vi "BonOMM-SAOMM.vi"() -> ()   [LabVIEW 2019] (continued)
                n1946 = local write "RangeTable"(FALSE ("RangeTable")) -> ()
                n1947 = case shown="Vrai" w5739 {
                  frame False {
                  }
                  frame True {
                    n1948 = local read "LimXPesto"() -> (w5740:dbl)
                    n1949 = local read "BrasPesto"() -> (w5741:bool)
                    n1950 = local read "Table VRN"() -> (w5750:refnum<visa-resource-name>)
                    n1951 = local read "Table Error"() -> (w5748:errorcluster)
                    n1952 = control-ref of="TERMINAL"() -> (w5753:refnum<vi>)
                    n1953 = control-ref of="Indicateur d'état"() -> (w5752:refnum<vi>)
                    n1954 = control-ref of="Table actif"() -> (w5745:refnum<vi>)
                    n1955 = call "Newmark-GotoAll.vi"("Table VRN IN"=w5750, "BrasPesto"=w5741, "Bool Refnum"=w5745, "LimXPesto"=w5740, "Notify?"=FALSE, "Error IN"=w5748, "Position X"="Rangement Y", "Position Y"="Rangement X", "Position Z"="Rangement Z") -> ("Table VRN OUT"=w5749:refnum<visa-resource-name>, "Error OUT"=w5747:errorcluster)  [unwired: 5 in]
                    n1956 = call "TERMINAL.vi"("Indicateur Refnum"=w5752, "Terminal Refnum"=w5753, "Indicateur d'état"="Commande de rangement des tables") -> ()
                    n1957 = local write "Table VRN"(w5749) -> ()
                    n1958 = local write "Table Error"(w5747) -> ()
                    n1959 = local write "Cible X"("Rangement Y") -> ()
                    n1960 = local write "Cible Y"("Rangement X") -> ()
                    n1961 = local write "Cible Z"("Rangement Z") -> ()
                  }
                }
              }
              event "GO": Value Change {
                n1962 = event-data() -> ()  [unwired: 1 in, 5 out]
                n1963 = flat-sequence {
                  frame #0 {
                    n1964 = control-ref of="TERMINAL"() -> (w5756:refnum<vi>)
                    n1965 = control-ref of="Indicateur d'état"() -> (w5755:refnum<vi>)
                    n1966 = local write "GO"(FALSE) -> ()
                    n1967 = call "TERMINAL.vi"("Indicateur Refnum"=w5755, "Terminal Refnum"=w5756, "Indicateur d'état"="Commande de déplacement du télescope") -> ()
                  }
                  frame #1 {
                    n1968 = local read "STATH"() -> (w5758:bool[])
                    n1969 = Index Array(array=w5758, index=7 ("Index")) -> (element=w5759:bool)
                    n1970 = case shown="Vrai" w5759 {
                      frame False {
                        w5761 = u32 0
                        # "Est-ce qu'on ne veut pas envoyez un stop à ce moment là ?"
                        n1971 = local read "FIFO d'erreur"() -> (w5763:T7)
                        n1972 = Bundle("TCS", w5761, w5761, "ATTENTION!!\nLes moteurs ne sont pas allumés.") -> (w5764:cluster{string, u32, u32, string})  [unwired: 1 in]
                        n1973 = Build Array (concatenate)(w5763, w5764) -> (w5762:T7)
                        n1974 = local write "FIFO d'erreur"(w5762) -> ()
                      }
                      frame True {
                        n1975 = control-ref of="TCS actif"() -> (w5767:refnum<vi>)
                        n1976 = local read "TCS VRN"() -> (w5768:refnum<visa-resource-name>)
                        n1977 = call "EXCOM-CMD.vi"("VRN IN"=w5768, "Bool Refnum"=w5767, "Commande #"=12) -> ("VRN OUT"=w5771:refnum<visa-resource-name>, "OK Done"=w5770:bool, "Error OUT"=w5769:errorcluster)  [unwired: 10 in]
                        n1978 = local write "TCS VRN"(w5771) -> ()
                        n1979 = local write "TCS Error"(w5769) -> ()
                        n1980 = case shown="Vrai" w5770 {
                          selector: w5770 -> [_ w5775]
                          frame False {
                            n1981 = One Button Dialog(message="ATTENTION!!\nProblème de communication\navec TCS-Ctrl", button name ("OK")="OK" ("nom du bouton (\"OK\")")) -> ()  [unwired: 1 out]
                          }
                          frame True {
                            "Déplacement usager" <- w5775
                          }
                        }
                      }
                    }
                  }
                }
              }
              event "Synctel": Value Change {
                n1982 = event-data() -> ()  [unwired: 1 in, 5 out]
                n1983 = local read "Mode Est"() -> (w5776:bool)
                n1984 = case shown="Faux" w5776 {
                  frame False {
                    n1985 = flat-sequence {
                      frame #0 {
                        n1986 = local write "Synctel"(FALSE) -> ()
                      }
                      frame #1 {
                        w5781 = ", " ("F button name (\"Cancel\")")
                        n1987 = local read "NO epoch"() -> (w5787:dbl)
                        n1988 = local read "N.O. A.D."() -> (w5783:string)
                        n1989 = local read "N.O. Déc."() -> (w5780:string)
                        n1990 = Number To Fractional String(number=w5787, width (-)=i16 6, precision (6)=i16 2) -> (F-format string=w5779:string)  [unwired: 1 in]
                        n1991 = Concatenate Strings("êtes vous certain de vouloir synchroniser \nles coordonnées de TCS sur :\nR.A. : " ("string"), w5783, "\nDEC : ", w5780, "\nEPOCH : ", w5779) -> (w5791:string)
                        n1992 = control-ref of="TERMINAL"() -> (w5785:refnum<vi>)
                        n1993 = control-ref of="Indicateur d'état"() -> (w5784:refnum<vi>)
                        n1994 = Concatenate Strings("Synchronisation sur : " ("Indicateur d'état"), w5783, w5781, w5780, w5781, w5779) -> (w5778:string)
                        n1995 = Two Button Dialog(message=w5791, 1:"NON" ("F button name (\"Cancel\")"), 2:"OUI" ("T button name (\"OK\")")) -> (T button?=w5793:bool)
                        n1996 = call "TERMINAL.vi"("Indicateur Refnum"=w5784, "Terminal Refnum"=w5785, "Indicateur d'état"=w5778) -> ()
                        n1997 = case shown="Vrai" w5793 {
                          tunnel: w5780 -> [_ w5807]
                          tunnel: w5783 -> [_ w5806]
                          frame False {
                          }
                          frame True {
                            # "Initialise RA et DEC\naux valeurs de Starry Night"
                            n1998 = local read "NO epoch"() -> (w5803:dbl)
                            n1999 = call "time-str-to-time-dbl-RA.vi"("Chaîne"=w5806) -> ("TCS_coords"=w5801:dbl)
                            n2000 = call "time-str-to-time-dbl-DEC.vi"("Chaîne"=w5807) -> ("TCS_coords"=w5802:dbl)
                            n2001 = control-ref of="TCS actif"() -> (w5796:refnum<vi>)
                            n2002 = local read "TCS VRN"() -> (w5804:refnum<visa-resource-name>)
                            n2003 = Build Array(w5801, w5802, w5803) -> (w5800:dbl[])
                            n2004 = call "EXCOM-CMD.vi"("VRN IN"=w5804, "Bool Refnum"=w5796, "Commande #"=3 ("NombredArguments"), "Args"=w5800) -> ("VRN OUT"=w5797:refnum<visa-resource-name>, "OK Done"=w5798:bool, "Error OUT"=w5799:errorcluster)  [unwired: 9 in]
                            n2005 = local write "TCS Error"(w5799) -> ()
                            n2006 = local write "TCS VRN"(w5797) -> ()
                            n2007 = case shown="Faux" w5798 {
                              frame False {
                                n2008 = One Button Dialog(message="ATTENTION!!\nLa commande SyncTEL a échoué.\nVérifiez TCS.", button name ("OK")="OK" ("nom du bouton (\"OK\")")) -> ()  [unwired: 1 out]
                              }
                              frame True {
                              }
                            }
                          }
                        }
                      }
                      frame #2 {
                        n2009 = control-ref of="TCS actif"() -> (w5810:refnum<vi>)
                        n2010 = local read "TCS VRN"() -> (w5812:refnum<visa-resource-name>)
                        n2011 = local read "TCS Error"() -> (w5811:errorcluster)
                        n2012 = call "EXCOM-CMD.vi"("VRN IN"=w5812, "Bool Refnum"=w5810, "Commande #"=13 ("NombredArguments"), "Error IN"=w5811) -> ("VRN OUT"=w5814:refnum<visa-resource-name>, "Error OUT"=w5813:errorcluster)  [unwired: 9 in, 1 out]
                        n2013 = local write "TCS VRN"(w5814) -> ()
                        n2014 = local write "TCS Error"(w5813) -> ()
                      }
                    }
                  }
                  frame True {
                    n2015 = One Button Dialog(message="Impossible de synchroniser les coordonnées en mode inversé.", button name ("OK")="Ok") -> ()  [unwired: 1 out]
                  }
                }
              }
              event "RotationTCS": Value Change {
                n2016 = event-data() -> ()  [unwired: 1 in, 5 out]
              }
              event "ModifRotation": Value Change {
                n2017 = event-data() -> ()  [unwired: 1 in, 5 out]
                n2018 = case shown="Vrai" "ModifRotation" {
                  frame False {
                  }
                  frame True {
                    n2019 = local read "RotationTCS"() -> (w5826:dbl)
                    n2020 = control-ref of="TCS actif"() -> (w5819:refnum<vi>)
                    n2021 = local read "TCS VRN"() -> (w5823:refnum<visa-resource-name>)
                    n2022 = call "Set rotation.vi"("Rot.In"=w5826) -> ("DONE"=w5825:bool, "Rot.Out"=w5824:dbl)
                    n2023 = case shown="Vrai" w5825 {
                      selector: w5825 -> [w5827 _]
                      tunnel: w5824 -> [_ w5830]
                      tunnel: w5823 -> [_ w5834]
                      tunnel: w5819 -> [_ w5833]
                      frame False {
                        n2024 = local write "ModifRotation"(w5827) -> ()
                      }
                      frame True {
                        n2025 = In Range and Coerce(upper limit=180.0, x=w5830, lower limit=0.0 ("upper limit")) -> (coerced(x)=w5828:dbl, In Range?=w5829:bool)
                        n2026 = case shown="Vrai" w5829 {
                          tunnel: w5834 -> [_ w5839]
                          tunnel: w5833 -> [_ w5838]
                          tunnel: w5828 -> [_ w5836]
                          frame False {
                            n2027 = One Button Dialog(message="Les valeurs envoyées doivent être comprises entre 0° et 180°") -> ()  [unwired: 1 in, 1 out]
                          }
                          frame True {
                            # "Bug TCS"
                            n2028 = expression code="90-x"(w5836) -> (w5837:dbl)
                            n2029 = stacked-sequence {
                              tunnel: w5837 -> [_ w5845 _]
                              tunnel: w5839 -> [_ w5849 _]
                              tunnel: w5838 -> [_ w5843 _]
                              frame #0 {
                                w5841 = 2
                                w5840 = 2
                                # "Attendre 0.5 sec afin que la boucle de surveillance se termine"
                                n2030 = property on="ModifRotation" class="Bool (strict)"("Blinking"=TRUE) -> ()  [unwired: 2 in, 2 out]
                                n2031 = property on="GO" class="Bool (strict)"("Disabled"=w5840) -> ()  [unwired: 2 in, 2 out]
                                n2032 = property on="ModCoor" class="Bool (strict)"("Disabled"=w5840) -> ()  [unwired: 2 in, 2 out]
                                n2033 = property on="Synctel" class="Bool (strict)"("Disabled"=w5840) -> ()  [unwired: 2 in, 2 out]
                                n2034 = property on="Offset OK" class="Bool (strict)"("Disabled"=w5840) -> ()  [unwired: 2 in, 2 out]
                                n2035 = property on="Zénith" class="Bool (strict)"("Disabled"=w5841) -> ()  [unwired: 2 in, 2 out]
                                n2036 = property on="Écran" class="Bool (strict)"("Disabled"=w5841) -> ()  [unwired: 2 in, 2 out]
                                n2037 = property on="ModifFoyer" class="Bool (strict)"("Disabled"=w5841) -> ()  [unwired: 2 in, 2 out]
                                n2038 = property on="Range" class="Bool (strict)"("Disabled"=w5841) -> ()  [unwired: 2 in, 2 out]
                                n2039 = property on="ModifDome" class="Bool (strict)"("Disabled"=w5841) -> ()  [unwired: 2 in, 2 out]
                                n2040 = property on="Coupole-Tél" class="Bool (strict)"("Disabled"=w5841) -> ()  [unwired: 2 in, 2 out]
                              }
                              frame #1 {
                                # "Changement de la \nposition du rotateur."
                                n2041 = Build Array(w5845) -> (w5846:dbl[])
                                n2042 = call "EXCOM-CMD.vi"("VRN IN"=w5849, "Bool Refnum"=w5843, "Commande #"=4, "Args"=w5846) -> ("VRN OUT"=w5847:refnum<visa-resource-name>, "OK Done"=w5850:bool, "Error OUT"=w5844:errorcluster)  [unwired: 9 in]
                                n2043 = case shown="Vrai" w5850 {
                                selector: w5850 -> [w5853 _]
                                tunnel: w5847 -> [w5851 w5867]
                                tunnel: w5844 -> [w5852 w5866]
                                tunnel: [w5852 w5865] -> _
                                tunnel: [w5851 w5864] -> _
                                tunnel: [w5853 w5863] -> _
                                tunnel: w5843 -> [_ w5862]
                                frame False {
                                w5854 = 4
                                n2044 = local read "CmdPending"() -> (w5855:bool)
                                n2045 = local read "FIFO d'erreur"() -> (w5859:T7)
                                n2046 = case shown="Vrai" w5855 {
                                tunnel: w5854 -> [_ w5861]
                                frame False {
                                }
                                frame True {
                                n2047 = local write "Error Code"(w5861) -> ()
                                }
                                }
                                n2048 = Bundle("ETCS", w5854, w5854, "ATTENTION !!!\nLa commande MODIF-ROTATION a échoué.\nRecommencez ou vérifiez TCS.") -> (w5858:cluster{string, i32, i32, string})  [unwired: 1 in]
                                n2049 = Build Array (concatenate)(w5859, w5858) -> (w5860:T7)
                                n2050 = local write "FIFO d'erreur"(w5860) -> ()
                                }
                                frame True {
                                n2051 = stacked-sequence {
                                tunnel: w5867 -> [_ w5877]
                                tunnel: w5866 -> [_ w5876]
                                tunnel: [_ w5873] -> w5865
                                tunnel: [_ w5872] -> w5864
                                tunnel: [_ w5871] -> w5863
                                tunnel: w5862 -> [_ w5869]
                                frame #0 {
                                # "Devrait probablement vérifier l'état du flag à la place ..."
                                # "attendre 600ms que la commande GO soit acceptée par TCS"
                                n2052 = Wait (ms)(milliseconds to wait=u32 600 ("attente (ms)")) -> ()  [unwired: 1 out]
                                }
                                frame #1 {
                                n2053 = Tick Count (ms)() -> (millisecond timer value=w5879:u32)
                                n2054 = while {
                                tunnel: w5879 -> [w5893]
                                tunnel: [w5890] -> w5878
                                tunnel: w5877 -> [w5885]
                                tunnel: w5876 -> [w5884]
                                tunnel: [w5883] -> w5875
                                tunnel: [w5882] -> w5874
                                tunnel: [w5881] -> w5870
                                tunnel: w5869 -> [w5880]
                                stop <- w5892 stop-if-true
                                # "Max 90 secondes"
                                # "Bit 1 = slew ON ou OFF"
                                n2055 = Tick Count (ms)() -> (millisecond timer value=w5894:u32)
                                n2056 = call "EXCOM-26.vi"("VRN IN"=w5885, "Bool Refnum"=w5880, "Error IN"=w5884) -> ("VRN OUT"=w5883:refnum<visa-resource-name>, "OK Done"=w5881:bool, "STATEX"=w5886:bool[], "Error OUT"=w5882:errorcluster)  [unwired: 6 in, 3 out]
                                n2057 = Wait Until Next ms Multiple(millisecond multiple=u32 500 ("n millisecondes")) -> ()  [unwired: 1 out]
                                n2058 = Subtract(x=w5894, y=w5893) -> (x-y=w5895:u32)
                                n2059 = Greater?(x=w5895, y=u32 90000) -> (0:w5890:bool)
                                n2060 = Index Array(array=w5886, index=1 ("Index")) -> (element=w5887:bool)
                                n2061 = Not(x=w5887) -> (.not. x?=w5889:bool)
                                n2062 = Or(x=w5889, y=w5890) -> (x .or. y?=w5892:bool)
                                }
                                n2063 = case shown="Vrai" w5878 {
                                tunnel: w5875 -> [w5898 w5905]
                                tunnel: w5874 -> [w5897 w5904]
                                tunnel: [w5897 w5903] -> w5873
                                tunnel: [w5898 w5902] -> w5872
                                tunnel: [w5899 w5901] -> w5871
                                tunnel: w5870 -> [w5899 _]
                                tunnel: w5869 -> [_ w5900]
                                frame False {
                                }
                                frame True {
                                w5912 = 4
                                n2064 = local read "CmdPending"() -> (w5906:bool)
                                n2065 = case shown="Vrai" w5906 {
                                tunnel: w5912 -> [_ w5914]
                                frame False {
                                }
                                frame True {
                                n2066 = local write "Error Code"(w5914) -> ()
                                }
                                }
                                n2067 = call "EXCOM-CMD.vi"("VRN IN"=w5905, "Bool Refnum"=w5900, "Commande #"=13 ("NombredArguments"), "Error IN"=w5904) -> ("VRN OUT"=w5902:refnum<visa-resource-name>, "OK Done"=w5901:bool, "Error OUT"=w5903:errorcluster)  [unwired: 9 in]
                                n2068 = local read "FIFO d'erreur"() -> (w5910:T7)
                                n2069 = Bundle("ETCS", w5912, w5912, "Le rotateur ne semble pas avoir atteint sa position") -> (w5909:cluster{string, i32, i32, string})  [unwired: 1 in]
                                n2070 = Build Array (concatenate)(w5910, w5909) -> (w5911:T7)
                                n2071 = local write "FIFO d'erreur"(w5911) -> ()
                                n2072 = case shown="Faux" w5901 {
                                frame False {
                                w5916 = 128
                                n2073 = local read "CmdPending"() -> (w5915:bool)
                                n2074 = case shown="Vrai" w5915 {
                                tunnel: w5916 -> [_ w5922]
                                frame False {
                                }
                                frame True {
                                n2075 = local write "Error Code"(w5922) -> ()
                                }
                                }
                                n2076 = local read "FIFO d'erreur"() -> (w5918:T7)
                                n2077 = Bundle("ETCS", w5916, w5916, "ATTENTION!!\nLa commande STOP a échoué.\nVérifiez TCS.") -> (w5919:cluster{string, i32, i32, string})  [unwired: 1 in]
                                n2078 = Build Array (concatenate)(w5918, w5919) -> (w5917:T7)
                                n2079 = local write "FIFO d'erreur"(w5917) -> ()
                                }
                                frame True {
                                }
                                }
                                }
                                }
                                }
                                }
                                }
                                }
                              }
                              frame #2 {
                                w5925 = 0
                                w5926 = 0
                                w5923 = FALSE
                                # "Voir le fonctionnement de \"CMDPENDING\""
                                n2080 = property on="ModifDome" class="Bool (strict)"("Disabled"=w5926) -> ()  [unwired: 2 in, 2 out]
                                n2081 = property on="Écran" class="Bool (strict)"("Disabled"=w5926) -> ()  [unwired: 2 in, 2 out]
                                n2082 = property on="Range" class="Bool (strict)"("Disabled"=w5926) -> ()  [unwired: 2 in, 2 out]
                                n2083 = property on="Zénith" class="Bool (strict)"("Disabled"=w5926) -> ()  [unwired: 2 in, 2 out]
                                n2084 = property on="Synctel" class="Bool (strict)"("Disabled"=w5926) -> ()  [unwired: 2 in, 2 out]
                                n2085 = property on="Offset OK" class="Bool (strict)"("Disabled"=w5926) -> ()  [unwired: 2 in, 2 out]
                                n2086 = local read "CmdPending"() -> (w5924:bool)
                                n2087 = property on="GO" class="Bool (strict)"("Disabled"=w5925) -> ()  [unwired: 2 in, 2 out]
                                n2088 = property on="ModCoor" class="Bool (strict)"("Disabled"=w5925) -> ()  [unwired: 2 in, 2 out]
                                n2089 = property on="ModifFoyer" class="Bool (strict)"("Disabled"=w5925) -> ()  [unwired: 2 in, 2 out]
                                n2090 = property on="Coupole-Tél" class="Bool (strict)"("Disabled"=w5925) -> ()  [unwired: 2 in, 2 out]
                                n2091 = case shown="Vrai" w5924 {
                                frame False {
                                }
                                frame True {
                                n2092 = local write "CmdPending"(FALSE) -> ()
                                }
                                }
                                n2093 = property on="ModifRotation" class="Bool (strict)"("Blinking"=w5923) -> ()  [unwired: 2 in, 2 out]
                                n2094 = local write "ModifRotation"(w5923) -> ()
                              }
                            }
                          }
                        }
                      }
                    }
                    n2095 = control-ref of="TERMINAL"() -> (w5822:refnum<vi>)
                    n2096 = control-ref of="Indicateur d'état"() -> (w5821:refnum<vi>)
                    n2097 = call "TERMINAL.vi"("Indicateur Refnum"=w5821, "Terminal Refnum"=w5822, "Indicateur d'état"="Modification de la rotation de la bonnette") -> ()
                  }
                }
              }
              event "ModifFoyer": Value Change {
                n2098 = event-data() -> ()  [unwired: 1 in, 5 out]
                n2099 = case shown="Vrai" "ModifFoyer" {
                  frame False {
                  }
                  frame True {
                    n2100 = control-ref of="TERMINAL"() -> (w5933:refnum<vi>)
                    n2101 = control-ref of="Indicateur d'état"() -> (w5932:refnum<vi>)
                    n2102 = local read "Foyer"() -> (w5930:dbl)
                    n2103 = control-ref of="TCS actif"() -> (w5929:refnum<vi>)
                    n2104 = local read "TCS VRN"() -> (w5936:refnum<visa-resource-name>)
                    n2105 = call "TERMINAL.vi"("Indicateur Refnum"=w5932, "Terminal Refnum"=w5933, "Indicateur d'état"="Modification logicielle du foyer") -> ()
                    n2106 = call "Set foyer.vi"("Foyer In"=w5930) -> ("Foyer Out"=w5935:dbl, "DONE"=w5937:bool, "sortie foyer sonde"=w5934:bool)  [unwired: 1 in]
                    n2107 = case shown="Vrai" w5937 {
                      selector: w5937 -> [w5938 _]
                      tunnel: w5935 -> [_ w5943]
                      tunnel: w5936 -> [_ w5942]
                      tunnel: w5934 -> [_ w5941]
                      tunnel: w5930 -> [_ w5940]
                      tunnel: w5929 -> [_ w5939]
                      frame False {
                        n2108 = local write "ModifFoyer"(w5938) -> ()
                      }
                      frame True {
                        n2109 = stacked-sequence {
                          tunnel: w5943 -> [_ w5948 _]
                          tunnel: w5942 -> [_ w5950 _]
                          tunnel: w5941 -> [_ w5949 _]
                          tunnel: w5940 -> [_ w5947 _]
                          tunnel: w5939 -> [_ w5946 _]
                          frame #0 {
                            w5945 = 2
                            n2110 = property on="GO" class="Bool (strict)"("Disabled"=w5945) -> ()  [unwired: 2 in, 2 out]
                            n2111 = property on="ModCoor" class="Bool (strict)"("Disabled"=w5945) -> ()  [unwired: 2 in, 2 out]
                            n2112 = property on="Synctel" class="Bool (strict)"("Disabled"=w5945) -> ()  [unwired: 2 in, 2 out]
                            n2113 = property on="Offset OK" class="Bool (strict)"("Disabled"=w5945) -> ()  [unwired: 2 in, 2 out]
                            n2114 = property on="Zénith" class="Bool (strict)"("Disabled"=w5945) -> ()  [unwired: 2 in, 2 out]
                            n2115 = property on="Écran" class="Bool (strict)"("Disabled"=w5945) -> ()  [unwired: 2 in, 2 out]
                            n2116 = property on="ModifRotation" class="Bool (strict)"("Disabled"=w5945) -> ()  [unwired: 2 in, 2 out]
                            n2117 = property on="Range" class="Bool (strict)"("Disabled"=w5945) -> ()  [unwired: 2 in, 2 out]
                            n2118 = property on="ModifDome" class="Bool (strict)"("Disabled"=w5945) -> ()  [unwired: 2 in, 2 out]
                            n2119 = property on="Coupole-Tél" class="Bool (strict)"("Disabled"=w5945) -> ()  [unwired: 2 in, 2 out]
                            n2120 = property on="ModifFoyer" class="Bool (strict)"("Blinking"=TRUE) -> ()  [unwired: 2 in, 2 out]
                          }
                          frame #1 {
                            n2121 = while {
                              tunnel: w5950 -> [w5966]
                              tunnel: w5949 -> [w5965]
                              tunnel: w5948 -> [w5964]
                              tunnel: w5947 -> [w5961]
                              tunnel: w5946 -> [w5951]
                              i -> [w5956]
                              stop <- w5957 stop-if-true
                              n2122 = flat-sequence {
                                tunnel: w5966 -> [w5976]
                                tunnel: w5965 -> [w5975]
                                tunnel: w5964 -> [w5972]
                                tunnel: [w5974] -> w5953
                                tunnel: w5951 -> [w5967]
                                tunnel: [w6060] -> w5960
                                frame #0 {
                                n2123 = Build Array(w5972) -> (w5973:dbl[])
                                n2124 = call "EXCOM-CMD.vi"("VRN IN"=w5976, "Bool Refnum"=w5967, "Commande #"=27 ("NombredArguments"), "Args"=w5973) -> ("VRN OUT"=w5971:refnum<visa-resource-name>, "OK Done"=w5978:bool, "Error OUT"=w5970:errorcluster)  [unwired: 9 in]
                                n2125 = case shown="Vrai" w5978 {
                                tunnel: w5971 -> [w5980 w5991]
                                tunnel: w5975 -> [_ w5990]
                                tunnel: w5972 -> [_ w5989]
                                tunnel: [TRUE w5988] -> w5974
                                tunnel: w5970 -> [w5979 w5987]
                                tunnel: [w5980 w5986] -> w5969
                                tunnel: [w5979 w5985] -> w5968
                                tunnel: w5967 -> [_ w5984]
                                frame False {
                                n2126 = One Button Dialog(message="ATTENTION!!\nLa commande MODIF-FOYER a échoué.\nRecommencez ou vérifiez TCS.", button name ("OK")="OK" ("nom du bouton (\"OK\")")) -> ()  [unwired: 1 out]
                                }
                                frame True {
                                n2127 = stacked-sequence {
                                tunnel: w5991 -> [_ w6002 _ _]
                                tunnel: w5990 -> [_ _ w6044 _]
                                tunnel: w5989 -> [_ _ w6045 _]
                                tunnel: [_ w6001 _ _] -> w5988
                                tunnel: w5987 -> [_ w6000 _ _]
                                tunnel: [_ w5997 _ _] -> w5986
                                tunnel: [_ w5996 _ _] -> w5985
                                tunnel: w5984 -> [_ w5994 _ _]
                                frame #0 {
                                # "Encore une fois, on devrait vérifier avec les bits d'états ..."
                                # "attendre 1s que la commande soit acceptée par TCS"
                                n2128 = Wait (ms)(milliseconds to wait=u32 1000 ("attente (ms)")) -> ()  [unwired: 1 out]
                                }
                                frame #1 {
                                # "Changement de  la valeur du foyer."
                                n2129 = Tick Count (ms)() -> (millisecond timer value=w6003:u32)
                                n2130 = while {
                                tunnel: w6003 -> [w6017]
                                tunnel: [w6014] -> w6001
                                tunnel: w6002 -> [w6009]
                                tunnel: w6000 -> [w6008]
                                tunnel: [w6007] -> w5999
                                tunnel: [w6006] -> w5998
                                tunnel: [w6005] -> w5995
                                tunnel: w5994 -> [w6004]
                                tunnel: [w6004] -> w5993
                                stop <- w6016 stop-if-true
                                n2131 = Tick Count (ms)() -> (millisecond timer value=w6018:u32)
                                n2132 = call "EXCOM-26.vi"("VRN IN"=w6009, "Bool Refnum"=w6004, "Error IN"=w6008) -> ("VRN OUT"=w6007:refnum<visa-resource-name>, "OK Done"=w6005:bool, "STATEX"=w6010:bool[], "Error OUT"=w6006:errorcluster)  [unwired: 6 in, 3 out]
                                n2133 = Subtract(x=w6018, y=w6017) -> (x-y=w6019:u32)
                                n2134 = Greater?(x=w6019, y=u32 180000) -> (0:w6014:bool)
                                n2135 = Index Array(array=w6010, index=0 ("Index")) -> (element=w6011:bool)
                                n2136 = Not(x=w6011) -> (.not. x?=w6013:bool)
                                n2137 = Or(x=w6013, y=w6014) -> (x .or. y?=w6016:bool)
                                n2138 = Wait Until Next ms Multiple(millisecond multiple=u32 500 ("n millisecondes")) -> ()  [unwired: 1 out]
                                }
                                n2139 = case shown="Vrai" w6001 {
                                tunnel: w5999 -> [w6022 w6028]
                                tunnel: w5998 -> [w6021 w6027]
                                tunnel: [w6022 w6026] -> w5997
                                tunnel: [w6021 w6025] -> w5996
                                tunnel: w5995 -> [_ w6024]
                                tunnel: w5993 -> [_ w6023]
                                frame False {
                                }
                                frame True {
                                n2140 = One Button Dialog(message="ATTENTION!!\nProblème d'ajustement\ndu foyer du télescope.\nVérifiez TCS.", button name ("OK")="OK" ("nom du bouton (\"OK\")")) -> (true=w6030:bool)
                                n2141 = case shown="Vrai" w6030 {
                                tunnel: w6028 -> [w6033 w6039]
                                tunnel: w6027 -> [w6032 w6038]
                                tunnel: [w6033 w6037] -> w6026
                                tunnel: [w6032 w6036] -> w6025
                                tunnel: w6024 -> [_ _]
                                tunnel: w6023 -> [_ w6034]
                                frame False {
                                }
                                frame True {
                                n2142 = call "EXCOM-CMD.vi"("VRN IN"=w6039, "Bool Refnum"=w6034, "Commande #"=13 ("NombredArguments"), "Error IN"=w6038) -> ("VRN OUT"=w6037:refnum<visa-resource-name>, "OK Done"=w6035:bool, "Error OUT"=w6036:errorcluster)  [unwired: 9 in]
                                n2143 = case shown="Faux" w6035 {
                                frame False {
                                n2144 = One Button Dialog(message="ATTENTION!!\nLa commande STOP a échoué.\nVérifiez TCS.", button name ("OK")="OK" ("nom du bouton (\"OK\")")) -> ()  [unwired: 1 out]
                                }
                                frame True {
                                n2145 = Wait (ms)(milliseconds to wait=u32 10 ("attente (ms)")) -> ()  [unwired: 1 out]
                                }
                                }
                                }
                                }
                                }
                                }
                                }
                                frame #2 {
                                n2146 = case shown="Vrai" w6044 {
                                tunnel: w6045 -> [_ w6058]
                                frame False {
                                }
                                frame True {
                                n2147 = formula code="foyersonde=foyertel*k1+k0;"("foyertel"=w6058, "k0"="k0_focus", "k1"="k1_focus") -> ("foyersonde"=w6048:dbl)
                                n2148 = local read "Position X"() -> (w6047:dbl)
                                n2149 = local read "Position Y"() -> (w6046:dbl)
                                n2150 = local read "CentreTel X"() -> (w6055:dbl)
                                n2151 = local read "CentreTel Y"() -> (w6054:dbl)
                                n2152 = local read "a1_focus"() -> (w6052:dbl)
                                n2153 = local read "a2_focus"() -> (w6051:dbl)
                                n2154 = local read "a3_focus"() -> (w6050:dbl)
                                n2155 = call "Calc_focus.vi"("Pos X"=w6047, "Pos Y"=w6046, "Cen X"=w6055, "Cen Y"=w6054, "a1"=w6052, "a2"=w6051, "a3"=w6050) -> ("Residu"=w6053:dbl)  [unwired: 7 in, 1 out]
                                n2156 = Subtract(x=w6048, y=w6053) -> (x-y=w6049:dbl)
                                n2157 = local write "FoyerAuCentre"(w6049) -> ()
                                }
                                }
                                }
                                frame #3 {
                                n2158 = Wait (ms)(milliseconds to wait=u32 750) -> ()  [unwired: 1 out]
                                }
                                }
                                }
                                }
                                n2159 = local write "TCS Error"(w5968) -> ()
                                n2160 = local write "TCS VRN"(w5969) -> ()
                                }
                                frame #1 {
                                n2161 = local read "Foyer"() -> (w6060:dbl)
                                }
                              }
                              n2162 = local read "Annulation du foyer"() -> (w5952:bool)
                              n2163 = Subtract(x=w5960, y=w5961) -> (x-y=w5963:dbl)
                              n2164 = Greater?(x=w5956, y=2) -> (0:w5954:bool)
                              n2165 = Absolute Value(x=w5963) -> (abs(x)=w5962:dbl)
                              n2166 = Greater?(x=w5962, y=1.0) -> (0:w5958:bool)
                              n2167 = Compound Arithmetic op=OR(w5958, w5954, w5953, w5952) -> (w5957:bool)
                            }
                          }
                          frame #2 {
                            w6062 = 0
                            w6061 = FALSE
                            n2168 = property on="ModifDome" class="Bool (strict)"("Disabled"=w6062) -> ()  [unwired: 2 in, 2 out]
                            n2169 = property on="Écran" class="Bool (strict)"("Disabled"=w6062) -> ()  [unwired: 2 in, 2 out]
                            n2170 = property on="Range" class="Bool (strict)"("Disabled"=w6062) -> ()  [unwired: 2 in, 2 out]
                            n2171 = property on="Zénith" class="Bool (strict)"("Disabled"=w6062) -> ()  [unwired: 2 in, 2 out]
                            n2172 = property on="Synctel" class="Bool (strict)"("Disabled"=w6062) -> ()  [unwired: 2 in, 2 out]
                            n2173 = property on="Offset OK" class="Bool (strict)"("Disabled"=w6062) -> ()  [unwired: 2 in, 2 out]
                            n2174 = property on="GO" class="Bool (strict)"("Disabled"=w6062) -> ()  [unwired: 2 in, 2 out]
                            n2175 = property on="ModCoor" class="Bool (strict)"("Disabled"=w6062) -> ()  [unwired: 2 in, 2 out]
                            n2176 = property on="ModifRotation" class="Bool (strict)"("Disabled"=w6062) -> ()  [unwired: 2 in, 2 out]
                            n2177 = property on="Coupole-Tél" class="Bool (strict)"("Disabled"=w6062) -> ()  [unwired: 2 in, 2 out]
                            n2178 = property on="ModifFoyer" class="Bool (strict)"("Blinking"=w6061) -> ()  [unwired: 2 in, 2 out]
                            n2179 = local write "Annulation du foyer"(w6061) -> ()
                            n2180 = local write "ModifFoyer"(w6061) -> ()
                          }
                        }
                      }
                    }
                  }
                }
              }
              event "ModifDome": Value Change {
                n2181 = event-data() -> ("NewVal"=w6063:bool)  [unwired: 1 in, 4 out]
                n2182 = case shown="Vrai" w6063 {
                  frame False {
                  }
                  frame True {
                    n2183 = local read "Coupole"() -> (w6064:dbl)
                    n2184 = Number To Decimal String(number=w6064) -> (decimal integer string=w6065:string)  [unwired: 1 in]
                    n2185 = call "Set dome.vi"("Dome In"=w6064) -> ("DONE"=w6071:bool, "Dome Out"=w6070:dbl)
                    n2186 = Concatenate Strings("Synchronisation de la coupole sur " ("string"), w6065) -> (w6067:string)
                    n2187 = case shown="Vrai" w6071 {
                      selector: w6071 -> [w6072 _]
                      tunnel: w6070 -> [_ w6073]
                      frame False {
                        n2188 = local write "ModifDome"(w6072) -> ()
                      }
                      frame True {
                        n2189 = stacked-sequence {
                          tunnel: w6073 -> [_ w6083 _]
                          frame #0 {
                            n2190 = control-ref of="TCS C actif"() -> (w6074:refnum<vi>)
                            n2191 = call "TCS-Wait4Flag.vi"("Raise Flag ?"=TRUE, "Ctl Refnum IN"=w6074) -> ()  [unwired: 8 in, 2 out]
                          }
                          frame #1 {
                            n2192 = control-ref of="TCS actif"() -> (w6076:refnum<vi>)
                            n2193 = local read "TCS VRN"() -> (w6082:refnum<visa-resource-name>)
                            n2194 = Build Array(w6083) -> (w6079:dbl[])
                            n2195 = call "EXCOM-CMD.vi"("VRN IN"=w6082, "Bool Refnum"=w6076, "Commande #"=2 ("NombredArguments"), "Args"=w6079) -> ("VRN OUT"=w6080:refnum<visa-resource-name>, "OK Done"=w6078:bool, "Error OUT"=w6077:errorcluster)  [unwired: 9 in]
                            n2196 = local write "TCS VRN"(w6080) -> ()
                            n2197 = local write "TCS Error"(w6077) -> ()
                            n2198 = case shown="Faux" w6078 {
                              selector: w6078 -> [w6084 w6088]
                              frame False {
                                n2199 = local write "ModifDome"(w6084) -> ()
                                n2200 = One Button Dialog(message="ATTENTION!!\nProblème d'ajustement\nde la position de la coupole.\nVérifiez TCS.", button name ("OK")="OK" ("nom du bouton (\"OK\")")) -> ()  [unwired: 1 out]
                              }
                              frame True {
                                n2201 = Not(x=w6088) -> (.not. x?=w6087:bool)
                                n2202 = local write "ModifDome"(w6087) -> ()
                              }
                            }
                          }
                          frame #2 {
                            n2203 = local write "TCS actif"(FALSE ("BONC-TCS")) -> ()
                          }
                        }
                      }
                    }
                    n2204 = control-ref of="TERMINAL"() -> (w6069:refnum<vi>)
                    n2205 = control-ref of="Indicateur d'état"() -> (w6068:refnum<vi>)
                    n2206 = call "TERMINAL.vi"("Indicateur Refnum"=w6068, "Terminal Refnum"=w6069, "Indicateur d'état"=w6067) -> ()
                  }
                }
              }
              event "Coupole-Tél": Value Change {
                n2207 = event-data() -> ()  [unwired: 1 in, 5 out]
                n2208 = Select(t="ON" ("string"), s="Coupole-Tél", f="OFF" ("string")) -> (s? t:f=w6099:string)
                n2209 = control-ref of="TERMINAL"() -> (w6103:refnum<vi>)
                n2210 = control-ref of="Indicateur d'état"() -> (w6102:refnum<vi>)
                n2211 = Concatenate Strings("AUTO DOME : " ("string"), w6099) -> (w6100:string)
                n2212 = call "TERMINAL.vi"("Indicateur Refnum"=w6102, "Terminal Refnum"=w6103, "Indicateur d'état"=w6100) -> ()
                n2213 = Boolean To (0,1)(Boolean="Coupole-Tél") -> (0, 1=w6105:i16)
                n2214 = To Double Precision Float(number=w6105) -> (double precision float=w6095:dbl)
                n2215 = Build Array(w6095) -> (w6094:dbl[])
                n2216 = control-ref of="TCS actif"() -> (w6090:refnum<vi>)
                n2217 = local read "TCS VRN"() -> (w6104:refnum<visa-resource-name>)
                n2218 = call "EXCOM-CMD.vi"("VRN IN"=w6104, "Bool Refnum"=w6090, "Commande #"=20 ("NombredArguments"), "Args"=w6094) -> ("VRN OUT"=w6093:refnum<visa-resource-name>, "OK Done"=w6091:bool, "Error OUT"=w6092:errorcluster)  [unwired: 9 in]
                n2219 = local write "TCS Error"(w6092) -> ()
                n2220 = local write "TCS VRN"(w6093) -> ()
                n2221 = case shown="Faux" w6091 {
                  frame False {
                    n2222 = One Button Dialog(message="ATTENTION!!\nLa commande DOME ON/OFF a échoué.\nVérifiez TCS.", button name ("OK")="OK" ("nom du bouton (\"OK\")")) -> ()  [unwired: 1 out]
                  }
                  frame True {
                  }
                }
              }
              event "Offset OK": Value Change {
                n2223 = event-data() -> ("NewVal"=w6109:bool)  [unwired: 1 in, 4 out]
                n2224 = case shown="Vrai" w6109 {
                  frame False {
                  }
                  frame True {
                    # "OFFSET en\nsecondes d'arc"
                    # "Commande OFFSET\nSlew Enable"
                    # "MX"
                    # "MY"
                    # "Y"
                    # "X"
                    # "DEC"
                    # "AD"
                    n2225 = stacked-sequence {
                      seq-local: [_ w6158 _] -> [_ _ w6174]
                      tunnel: "Offset DEC" -> [w6121 w6156 _]
                      tunnel: "Offset RA" -> [w6112 w6157 _]
                      frame #0 {
                        n2226 = local read "XReference"() -> (w6114:dbl)
                        n2227 = Number To Fractional String(number=w6121, precision (6)=i16 2) -> (F-format string=w6117:string)  [unwired: 2 in]
                        n2228 = Number To Fractional String(number=w6112, precision (6)=i16 2) -> (F-format string=w6119:string)  [unwired: 2 in]
                        n2229 = Add(x=w6114, y=w6112) -> (x+y=w6113:dbl)
                        n2230 = Concatenate Strings("Envoi manuel d'un offset de " ("string"), w6119, ", " ("string"), w6117) -> (w6116:string)
                        n2231 = local write "XReference"(w6113) -> ()
                        n2232 = local write "Offset OK"(FALSE) -> ()
                        n2233 = control-ref of="TERMINAL"() -> (w6124:refnum<vi>)
                        n2234 = control-ref of="Indicateur d'état"() -> (w6125:refnum<vi>)
                        n2235 = call "TERMINAL.vi"("Indicateur Refnum"=w6125, "Terminal Refnum"=w6124, "Indicateur d'état"=w6116) -> ()
                        "Offset en cours" <- TRUE ("Offset en cours")
                      }
                      frame #1 {
                        n2236 = control-ref of="Mode"() -> (w6143:refnum<vi>)
                        n2237 = control-ref of="BrasPesto"() -> (w6128:refnum<vi>)
                        n2238 = control-ref of="SNR"() -> (w6131:refnum<vi>)
                        n2239 = control-ref of="LimXPesto"() -> (w6127:refnum<vi>)
                        n2240 = control-ref of="Position Z"() -> (w6149:refnum<vi>)
                        n2241 = control-ref of="DiffX"() -> (w6144:refnum<vi>)
                        n2242 = control-ref of="DiffY"() -> (w6145:refnum<vi>)
                        n2243 = control-ref of="MovingXY"() -> (w6130:refnum<vi>)
                        n2244 = control-ref of="TCS actif"() -> (w6151:refnum<vi>)
                        n2245 = control-ref of="Table actif"() -> (w6150:refnum<vi>)
                        n2246 = control-ref of="StartServo"() -> (w6148:refnum<vi>)
                        n2247 = control-ref of="Servo"() -> (w6147:refnum<vi>)
                        n2248 = control-ref of="StopServo"() -> (w6146:refnum<vi>)
                        n2249 = local read "TableAstrom"() -> (w6140:T4)
                        n2250 = local read "FieldAstrom"() -> (w6142:T4)
                        n2251 = local read "GuiderAstrom"() -> (w6141:T4)
                        n2252 = local read "TCS VRN"() -> (w6139:refnum<visa-resource-name>)
                        n2253 = local read "TCS Error"() -> (w6138:errorcluster)
                        n2254 = local read "Table VRN"() -> (w6137:refnum<visa-resource-name>)
                        n2255 = local read "Table Error"() -> (w6136:errorcluster)
                        n2256 = Bundle("TableAstrom"=w6140, "FieldAstrom"=w6142, "GuiderAstrom"=w6141) -> (w6134:T41)  [unwired: 1 in]
                        n2257 = Bundle("TCS VRN"=w6139, "TCS Error"=w6138, "Table VRN"=w6137, "Table Error"=w6136) -> (w6133:T42)  [unwired: 1 in]
                        n2258 = Bundle("TCS actif"=w6151, "Table actif"=w6150, "Position Z"=w6149, "StartServo"=w6148, "Mode"=w6143, "Servo"=w6147, "StopServo"=w6146, "DiffX"=w6144, "DiffY"=w6145, "SNR"=w6131, "MovingXY"=w6130, "BrasPesto"=w6128, "LimXPesto"=w6127) -> (w6135:T43)  [unwired: 1 in]
                        n2259 = local read "OffsetAcc"() -> (w6132:dbl)
                        n2260 = while {
                          tunnel: [FALSE] -> w6129
                          stop <- w6161 continue-if-true
                          n2261 = local read "enfoncé"() -> (w6163:bool)
                          n2262 = Wait (ms)(milliseconds to wait=u32 200) -> ()  [unwired: 1 out]
                          n2263 = Not(x=w6163) -> (.not. x?=w6162:bool)
                          n2264 = local write "enfoncé"(w6162) -> ()
                          n2265 = local read "Offset en cours"() -> (w6161:bool)
                        }
                        n2266 = call "Cheesy_Offset.vi"("Communications_Cluster"=w6133, "Astrom_Cluster"=w6134, "RA offset"=w6157, "DEC offset"=w6156, "VariablesReferences"=w6135, "OffsetAccuracy (pixels)"=w6132) -> ("Error code"=w6155:u8, "Undo offset"=w6158:bool, "Warning code"=w6154:u8)  [unwired: 6 in, 1 out]
                        n2267 = To Unsigned Long Integer(number=w6154) -> (unsigned 32bit integer=w6152:u32)
                        n2268 = To Unsigned Long Integer(number=w6155) -> (unsigned 32bit integer=w6153:u32)
                        n2269 = flat-sequence {
                          tunnel: w6153 -> [w6167]
                          tunnel: w6152 -> [w6166]
                          frame #0 {
                            w6168 = u32 0 ("Error Code IN")
                            n2270 = local read "FIFO d'erreur"() -> (w6165:T7)
                            n2271 = call "Error_Format.vi"("FIFO IN"=w6165, "Error Code IN"=w6168, "Warning Code IN"=w6168, "Error Bit"=w6167, "Warning Bit"=w6166, "Source"="offset") -> ("FIFO OUT"=w6164:T7)  [unwired: 11 in, 2 out]
                            n2272 = local write "FIFO d'erreur"(w6164) -> ()
                          }
                          frame #1 {
                            n2273 = local write "Offset en cours"(FALSE ("Offset en cours")) -> ()
                          }
                        }
                        n2274 = local write "enfoncé"(w6129) -> ()
                      }
                      frame #2 {
                        w6175 = FALSE
                        # "Utile ?"
                        n2275 = disable-structure shown="Disabled" {
                          frame Disabled {
                            n2276 = local read "Table VRN"() -> (w6178:refnum<visa-resource-name>)
                            n2277 = local read "Table Error"() -> (w6177:errorcluster)
                            n2278 = control-ref of="Table actif"() -> (w6176:refnum<vi>)
                            n2279 = call "Newmark-Stop.vi"("Table VRN IN"=w6178, "Bool Refnum"=w6176, "Error IN"=w6177) -> ("Table VRN OUT"=w6180:refnum<visa-resource-name>, "Error OUT"=w6179:errorcluster)  [unwired: 11 in]
                            n2280 = local write "Table Error"(w6179) -> ()
                            n2281 = local write "Table VRN"(w6180) -> ()
                          }
                          frame Enabled {
                          }
                        }
                        n2282 = local write "RangeTable"(w6175) -> ()
                        n2283 = local write "Calibration"(w6175) -> ()
                        n2284 = local write "stoptable"(w6175) -> ()
                        n2285 = local write "Alacible"(w6175) -> ()
                        n2286 = local write "Origine"(w6175) -> ()
                        n2287 = local write "Centre"(w6175) -> ()
                        n2288 = case shown="Faux" w6174 {
                          tunnel: [" : réussi" " : échoué"] -> w6172
                          frame False {
                          }
                          frame True {
                          }
                        }
                        n2289 = local read "TERMINAL"() -> (w6173:string)
                        n2290 = Concatenate Strings(w6173, w6172) -> (w6171:string)
                        n2291 = local write "TERMINAL"(w6171) -> ()
                      }
                    }
                  }
                }
              }
              event "ChoixFiltre": Value Change {
                n2292 = event-data() -> ()  [unwired: 1 in, 5 out]
                n2293 = local read "MC-BonOMM VRN"() -> (w6183:refnum<visa-resource-name>)
                n2294 = stacked-sequence {
                  seq-local: [w6191 _ _ _] -> [_ w6254 _ _]
                  seq-local: [w6199 _ _ _] -> [_ w6251 _ _]
                  tunnel: w6183 -> [_ w6253 _ w6300]
                  frame #0 {
                    w6203 = 2
                    n2295 = local read "F#"() -> (w6189:i32)
                    n2296 = Number To Decimal String(number=w6189) -> (decimal integer string=w6190:string)  [unwired: 1 in]
                    n2297 = control-ref of="TERMINAL"() -> (w6195:refnum<vi>)
                    n2298 = control-ref of="Indicateur d'état"() -> (w6196:refnum<vi>)
                    n2299 = Unbundle("ChoixFiltre") -> ("filtre #1"=w6206:bool, "filtre #2"=w6207:bool, "filtre #3"=w6208:bool, "filtre #4"=w6209:bool, "filtre #5"=w6210:bool, "filtre #6"=w6211:bool)
                    n2300 = Build Array(w6206, w6207, w6208, w6209, w6210, w6211) -> (w6212:bool[])
                    n2301 = Search 1D Array(1D array=w6212, element=TRUE) -> (index of element=w6197:i32)  [unwired: 1 in]
                    n2302 = Increment(x=w6197) -> (x+1=w6191:i32)
                    n2303 = Number To Decimal String(number=w6191) -> (decimal integer string=w6192:string)  [unwired: 1 in]
                    n2304 = Concatenate Strings("Passage du filtre #", w6190, " au filtre #", w6192) -> (w6188:string)
                    n2305 = call "TERMINAL.vi"("Indicateur Refnum"=w6196, "Terminal Refnum"=w6195, "Indicateur d'état"=w6188) -> ()
                    n2306 = Not Equal To 0?(x=w6191) -> (x != 0?=w6198:bool)
                    n2307 = property on="ChoixFiltre" class="Clust (strict)"() -> ("Controls[]"=w6202:refnum<vi>[])  [unwired: 2 in, 2 out]
                    n2308 = case shown="Vrai" w6198 {
                      selector: w6198 -> [w6236 _]
                      tunnel: w6197 -> [_ w6239]
                      tunnel: [w6236 w6238] -> w6199
                      frame False {
                      }
                      frame True {
                        n2309 = local read "Bypass Tech"() -> (w6237:bool)
                        n2310 = case shown="Vrai" w6237 {
                          selector: w6237 -> [_ w6249]
                          tunnel: w6239 -> [w6247 _]
                          tunnel: [w6240 w6249] -> w6238
                          frame False {
                            n2311 = local read "Tableau des filtres"() -> (w6248:string[])
                            n2312 = Index Array(array=w6248, index=w6247) -> (element=w6246:string)
                            n2313 = Concatenate Strings("Désirez-vous passer au filtre " ("message"), w6246, " ?" ("message")) -> (w6243:string)
                            n2314 = Two Button Dialog(message=w6243, 1:"NON" ("F button name (\"Cancel\")"), 2:"OUI" ("T button name (\"OK\")")) -> (T button?=w6240:bool)
                          }
                          frame True {
                          }
                        }
                      }
                    }
                    n2315 = Index Array(array=w6202, index=w6197) -> (element=w6201:refnum<vi>)
                    n2316 = property class="Cmde"(reference=w6201, "Blinking"=TRUE) -> ()  [unwired: 1 in, 2 out]
                    n2317 = Index Array(array=w6202, index #1=0 ("indice"), index #2=1 ("indice"), index #3=2 ("indice"), index #4=3 ("indice"), index #5=4 ("indice"), index #6=5 ("indice")) -> (element #1=w6214:refnum<vi>, element #2=w6215:refnum<vi>, element #3=w6216:refnum<vi>, element #4=w6217:refnum<vi>, element #5=w6218:refnum<vi>, element #6=w6219:refnum<vi>)
                    n2318 = property class="Cmde"(reference=w6214, "Disabled"=w6203) -> ()  [unwired: 1 in, 2 out]
                    n2319 = property class="Cmde"(reference=w6215, "Disabled"=w6203) -> ()  [unwired: 1 in, 2 out]
                    n2320 = property class="Cmde"(reference=w6216, "Disabled"=w6203) -> ()  [unwired: 1 in, 2 out]
                    n2321 = property class="Cmde"(reference=w6217, "Disabled"=w6203) -> ()  [unwired: 1 in, 2 out]
                    n2322 = property class="Cmde"(reference=w6218, "Disabled"=w6203) -> ()  [unwired: 1 in, 2 out]
                    n2323 = property class="Cmde"(reference=w6219, "Disabled"=w6203) -> ()  [unwired: 1 in, 2 out]
                    n2324 = local read "Tableau des filtres"() -> (w6187:string[])
                    n2325 = Current VI's Menubar() -> (w6184:refnum<k9>)
                    n2326 = for {
                      tunnel: w6187 -> [w6228] mode=indexing
                      tunnel: "@@" -> [w6232]
                      tunnel: "raf_" -> [w6233]
                      tunnel: w6184 -> [w6229]
                      tunnel: [w6227] -> _ mode=indexing
                      i -> [w6234]
                      n2327 = Number To Decimal String(number=w6234, width (-)=i16 1) -> (decimal integer string=w6231:string)
                      n2328 = Concatenate Strings(w6233, w6228, w6232, w6231) -> (w6230:string)
                      n2329 = Set Menu Item Info(6:FALSE ("checked"), 7:w6230, 9:TRUE ("enabled"), 10:w6228, 11:w6229) -> (0:w6227:errorcluster)  [unwired: 2 in, 1 out]
                    }
                  }
                  frame #1 {
                    n2330 = Not Equal To 0?(x=w6254) -> (x != 0?=w6252:bool)
                    n2331 = And(x=w6252, y=w6251) -> (x .and. y?=w6250:bool)
                    n2332 = case shown="Vrai" w6250 {
                      tunnel: w6254 -> [_ w6255]
                      tunnel: w6253 -> [_ w6256]
                      frame False {
                      }
                      frame True {
                        n2333 = Number To Decimal String(number=w6255, width (-)=i16 1) -> (decimal integer string=w6257:string)
                        n2334 = VISA Write(VISA resource name=w6256, write buffer=w6257) -> (VISA resource name out=w6258:refnum<visa-resource-name>)  [unwired: 1 in, 2 out]
                        n2335 = while {
                          tunnel: w6258 -> [w6268]
                          tunnel: w6255 -> [w6267]
                          stop <- w6266 stop-if-true
                          n2336 = while {
                            tunnel: w6268 -> [w6279]
                            tunnel: [w6278] -> w6263
                            tunnel: [w6277] -> w6261
                            i -> [w6282]
                            stop <- w6275 stop-if-true
                            n2337 = local read "Annulation en cours"() -> (w6274:bool)
                            n2338 = property class="Instr"(reference=w6279) -> (reference out=w6278:refnum<visa-resource-name>, "Serial Settings:Number of Bytes at Serial Port"=w6283:u32)  [unwired: 1 in, 1 out]
                            n2339 = Not Equal To 0?(x=w6283) -> (x != 0?=w6277:bool)
                            n2340 = call "Max-iteration.vi"("i max"=100, "i act"=w6282, "Valeur entrante"=w6277) -> ("break ?"=w6276:bool)
                            n2341 = Or(x=w6274, y=w6276) -> (x .or. y?=w6275:bool)
                            n2342 = Wait Until Next ms Multiple(millisecond multiple=u32 100) -> ()  [unwired: 1 out]
                          }
                          n2343 = case shown="Vrai" w6261 {
                            tunnel: w6263 -> [_ w6273]
                            tunnel: [0 w6270] -> w6262
                            frame False {
                            }
                            frame True {
                              n2344 = VISA Read(VISA resource name=w6273, byte count=u32 1) -> (read buffer=w6271:string)  [unwired: 1 in, 3 out]
                              n2345 = Decimal String To Number(string=w6271) -> (number=w6270:i32)  [unwired: 2 in, 1 out]
                            }
                          }
                          n2346 = Not(x=w6261) -> (.not. x?=w6265:bool)
                          n2347 = local write "F#"(w6262) -> ()
                          n2348 = Equal?(x=w6262, y=w6267) -> (x = y?=w6260:bool)
                          n2349 = local read "Annulation en cours"() -> (w6264:bool)
                          n2350 = Compound Arithmetic op=OR(w6260, w6265, w6264) -> (w6266:bool)
                        }
                      }
                    }
                  }
                  frame #2 {
                    n2351 = local read "Annulation en cours"() -> (w6284:bool)
                    n2352 = case shown="Faux" w6284 {
                      frame False {
                        n2353 = local read "MC_connect"() -> (w6285:bool)
                        n2354 = Wait (ms)(milliseconds to wait=u32 500) -> ()  [unwired: 1 out]
                        n2355 = case shown="Faux" w6285 {
                          frame False {
